vi "大富翁.vi"() -> ()   [LabVIEW 2014] (continued)
                      frame 4 {
                        n2785 = local read "玩家四財產"() -> (w2209:dbl)
                      }
                    }
                    n2786 = call "各種價格.vi"("Numeric"=w2178) -> ("買空地"=w2176:dbl)  [unwired: 4 in, 5 out]
                    n2787 = Greater Or Equal?(x=w2177, y=w2176) -> (x >= y?=w2175:bool)
                    n2788 = case shown="True" w2175 {
                      tunnel: w2178 -> [_ w2180]
                      frame False {
                        # "錢不夠"
                        n2789 = call "錢不夠.vi"() -> ()  [unwired: 4 in]
                      }
                      frame True {
                        # "錢夠"
                        n2790 = local read "換誰?"() -> (w2181:dbl)
                        n2791 = case shown="3" w2181 {
                          selector: w2181 -> [w2185 w2191 w2197 w2203]
                          tunnel: w2180 -> [w2184 w2190 w2196 w2202]
                          frame 1, Default {
                            # "誰買了地"
                            n2792 = call "各種價格.vi"("Numeric"=w2184) -> ("買空地"=w2183:dbl)  [unwired: 4 in, 5 out]
                            n2793 = local read "玩家一財產"() -> (w2187:dbl)
                            n2794 = Subtract(x=w2187, y=w2183) -> (x-y=w2186:dbl)
                            n2795 = local write "玩家一財產"(w2186) -> ()
                            n2796 = call "數字轉顏色.vi"("數字"=w2185) -> ("顏色數字"=w2182:dbl)  [unwired: 2 in]
                            n2797 = local write "17¾Á¤B"(w2182) -> ()
                            n2798 = local write "墾丁所有"(w2182) -> ()
                          }
                          frame 2 {
                            # "誰買了地"
                            n2799 = call "各種價格.vi"("Numeric"=w2190) -> ("買空地"=w2189:dbl)  [unwired: 4 in, 5 out]
                            n2800 = local read "玩家二財產"() -> (w2193:dbl)
                            n2801 = Subtract(x=w2193, y=w2189) -> (x-y=w2192:dbl)
                            n2802 = local write "玩家二財產"(w2192) -> ()
                            n2803 = call "數字轉顏色.vi"("數字"=w2191) -> ("顏色數字"=w2188:dbl)  [unwired: 2 in]
                            n2804 = local write "17¾Á¤B"(w2188) -> ()
                            n2805 = local write "墾丁所有"(w2188) -> ()
                          }
                          frame 3 {
                            # "誰買了地"
                            n2806 = local read "玩家三財產"() -> (w2198:dbl)
                            n2807 = call "各種價格.vi"("Numeric"=w2196) -> ("買空地"=w2195:dbl)  [unwired: 4 in, 5 out]
                            n2808 = Subtract(x=w2198, y=w2195) -> (x-y=w2199:dbl)
                            n2809 = call "數字轉顏色.vi"("數字"=w2197) -> ("顏色數字"=w2194:dbl)  [unwired: 2 in]
                            n2810 = local write "玩家三財產"(w2199) -> ()
                            n2811 = local write "17¾Á¤B"(w2194) -> ()
                            n2812 = local write "墾丁所有"(w2194) -> ()
                          }
                          frame 4 {
                            # "誰買了地"
                            n2813 = call "各種價格.vi"("Numeric"=w2202) -> ("買空地"=w2201:dbl)  [unwired: 4 in, 5 out]
                            n2814 = local read "玩家四財產"() -> (w2205:dbl)
                            n2815 = Subtract(x=w2205, y=w2201) -> (x-y=w2204:dbl)
                            n2816 = local write "玩家四財產"(w2204) -> ()
                            n2817 = call "數字轉顏色.vi"("數字"=w2203) -> ("顏色數字"=w2200:dbl)  [unwired: 2 in]
                            n2818 = local write "17¾Á¤B"(w2200) -> ()
                            n2819 = local write "墾丁所有"(w2200) -> ()
                          }
                        }
                      }
                    }
                  }
                }
              }
            }
          }
          frame 18 {
            n2820 = local read "屏東縣所有"() -> (w2210:u32)
            n2821 = Equal?(x=w2210, y=u32 16777215) -> (x = y?=w2213:bool)
            n2822 = case shown="True" w2213 {
              tunnel: w2212 -> [w2236 w2274]
              tunnel: [w2226 FALSE] -> w2211
              frame False {
                # "有主地"
                n2823 = local read "換誰?"() -> (w2229:dbl)
                n2824 = local read "屏東縣所有"() -> (w2217:u32)
                n2825 = call "數字轉顏色.vi"("數字"=w2229) -> ("顏色數字"=w2240:dbl)  [unwired: 2 in]
                n2826 = case shown="4" w2229 {
                  tunnel: [w2269 w2270 w2271 w2272] -> w2235
                  frame 1, Default {
                    n2827 = local read "玩家一財產"() -> (w2269:dbl)
                  }
                  frame 2 {
                    n2828 = local read "玩家二財產"() -> (w2270:dbl)
                  }
                  frame 3 {
                    n2829 = local read "玩家三財產"() -> (w2271:dbl)
                  }
                  frame 4 {
                    n2830 = local read "玩家四財產"() -> (w2272:dbl)
                  }
                }
                n2831 = Equal?(x=w2217, y=w2240) -> (x = y?=w2239:bool)
                n2832 = local read "18旅4"() -> (w2218:bool)
                n2833 = local read "18旅3"() -> (w2219:bool)
                n2834 = local read "18旅2"() -> (w2220:bool)
                n2835 = local read "18旅1"() -> (w2221:bool)
                n2836 = local read "18房4"() -> (w2222:bool)
                n2837 = local read "18房3"() -> (w2223:bool)
                n2838 = local read "18房2"() -> (w2224:bool)
                n2839 = local read "18房1"() -> (w2225:bool)
                n2840 = local read "屏東縣所有"() -> (w2216:u32)
                n2841 = call "房子數量.vi"("房子 1"=w2225, "房子 2"=w2224, "房子 3"=w2223, "房子 4"=w2222, "旅館 1"=w2221, "旅館 2"=w2220, "旅館 3"=w2219, "旅館 4"=w2218) -> ("房子數"=w2238:dbl, "旅館數"=w2237:dbl)  [unwired: 18 in]
                n2842 = call "顏色轉數字.vi"("顏色數字"=w2216) -> ("數字"=w2227:dbl)  [unwired: 2 in]
                n2843 = case shown="1, Default" w2227 {
                  tunnel: [w2245 w2246 w2247 w2248] -> w2231
                  frame 1, Default {
                    n2844 = local read "玩家一財產"() -> (w2245:dbl)
                  }
                  frame 2 {
                    n2845 = local read "玩家二財產"() -> (w2246:dbl)
                  }
                  frame 3 {
                    n2846 = local read "玩家三財產"() -> (w2247:dbl)
                  }
                  frame 4 {
                    n2847 = local read "玩家四財產"() -> (w2248:dbl)
                  }
                }
                n2848 = call "走到地.vi"("房子數量"=w2238, "自己的地?"=w2239, "旅館數量"=w2237, "編號"=w2236, "走到人財產"=w2235) -> ("走到人-?"=w2234:dbl, "蓋第幾棟"=w2232:dbl, "地主+?"=w2230:dbl, "破產?"=w2226:bool)
                n2849 = Subtract(x=w2235, y=w2234) -> (x-y=w2233:dbl)
                n2850 = Add(x=w2230, y=w2231) -> (x+y=w2228:dbl)
                n2851 = case shown="1, Default" w2227 {
                  tunnel: w2228 -> [w2241 w2242 w2243 w2244]
                  frame 1, Default {
                    n2852 = local write "玩家一財產"(w2241) -> ()
                  }
                  frame 2 {
                    n2853 = local write "玩家二財產"(w2242) -> ()
                  }
                  frame 3 {
                    n2854 = local write "玩家三財產"(w2243) -> ()
                  }
                  frame 4 {
                    n2855 = local write "玩家四財產"(w2244) -> ()
                  }
                }
                n2856 = case shown="6" w2232 {
                  frame 0, Default {
                  }
                  frame 1 {
                    n2857 = flat-sequence {
                      frame #0 {
                        n2858 = local write "18房1"(TRUE ("1房1")) -> ()
                      }
                      frame #1 {
                        n2859 = property on="18房1" class="Bool (strict)"("Visible"=TRUE) -> ()  [unwired: 2 in, 2 out]
                      }
                    }
                  }
                  frame 2 {
                    n2860 = flat-sequence {
                      frame #0 {
                        n2861 = local write "18房2"(TRUE ("1房2")) -> ()
                      }
                      frame #1 {
                        n2862 = property on="18房2" class="Bool (strict)"("Visible"=TRUE ("1房2")) -> ()  [unwired: 2 in, 2 out]
                      }
                    }
                  }
                  frame 3 {
                    n2863 = flat-sequence {
                      frame #0 {
                        n2864 = local write "18房3"(TRUE) -> ()
                      }
                      frame #1 {
                        n2865 = property on="18房3" class="Bool (strict)"("Visible"=TRUE) -> ()  [unwired: 2 in, 2 out]
                      }
                    }
                  }
                  frame 4 {
                    n2866 = flat-sequence {
                      frame #0 {
                        n2867 = local write "18房4"(TRUE) -> ()
                      }
                      frame #1 {
                        n2868 = property on="18房4" class="Bool (strict)"("Visible"=TRUE) -> ()  [unwired: 2 in, 2 out]
                      }
                    }
                  }
                  frame 5 {
                    n2869 = flat-sequence {
                      frame #0 {
                        n2870 = local write "18旅1"(TRUE) -> ()
                      }
                      frame #1 {
                        n2871 = property on="18旅1" class="Bool (strict)"("Visible"=TRUE) -> ()  [unwired: 2 in, 2 out]
                      }
                    }
                  }
                  frame 6 {
                    n2872 = flat-sequence {
                      frame #0 {
                        n2873 = local write "18旅2"(TRUE) -> ()
                      }
                      frame #1 {
                        n2874 = property on="18旅2" class="Bool (strict)"("Visible"=TRUE) -> ()  [unwired: 2 in, 2 out]
                      }
                    }
                  }
                  frame 7 {
                    n2875 = flat-sequence {
                      frame #0 {
                        n2876 = local write "18旅3"(TRUE) -> ()
                      }
                      frame #1 {
                        n2877 = property on="18旅3" class="Bool (strict)"("Visible"=TRUE) -> ()  [unwired: 2 in, 2 out]
                      }
                    }
                  }
                  frame 8 {
                    n2878 = flat-sequence {
                      frame #0 {
                        n2879 = local write "18旅4"(TRUE) -> ()
                      }
                      frame #1 {
                        n2880 = property on="18旅4" class="Bool (strict)"("Visible"=TRUE) -> ()  [unwired: 2 in, 2 out]
                      }
                    }
                  }
                }
                n2881 = case shown="1, Default" w2229 {
                  tunnel: w2233 -> [w2265 w2266 w2267 w2268]
                  frame 1, Default {
                    n2882 = local write "玩家一財產"(w2265) -> ()
                  }
                  frame 2 {
                    n2883 = local write "玩家二財產"(w2266) -> ()
                  }
                  frame 3 {
                    n2884 = local write "玩家三財產"(w2267) -> ()
                  }
                  frame 4 {
                    n2885 = local write "玩家四財產"(w2268) -> ()
                  }
                }
              }
              frame True {
                # "無主地"
                n2886 = call "購買土地.vi"() -> ("確定 2"=w2275:bool)  [unwired: 3 in]
                n2887 = case shown="True" w2275 {
                  tunnel: w2274 -> [_ w2279]
                  frame False {
                    # "不買"
                  }
                  frame True {
                    # "要買"
                    n2888 = local read "換誰?"() -> (w2280:dbl)
                    n2889 = case shown="4" w2280 {
                      tunnel: [w2307 w2308 w2309 w2310] -> w2278
                      frame 1, Default {
                        n2890 = local read "玩家一財產"() -> (w2307:dbl)
                      }
                      frame 2 {
                        n2891 = local read "玩家二財產"() -> (w2308:dbl)
                      }
                      frame 3 {
                        n2892 = local read "玩家三財產"() -> (w2309:dbl)
                      }
                      frame 4 {
                        n2893 = local read "玩家四財產"() -> (w2310:dbl)
                      }
                    }
                    n2894 = call "各種價格.vi"("Numeric"=w2279) -> ("買空地"=w2277:dbl)  [unwired: 4 in, 5 out]
                    n2895 = Greater Or Equal?(x=w2278, y=w2277) -> (x >= y?=w2276:bool)
                    n2896 = case shown="True" w2276 {
                      tunnel: w2279 -> [_ w2281]
                      frame False {
                        # "錢不夠"
                        n2897 = call "錢不夠.vi"() -> ()  [unwired: 4 in]
                      }
                      frame True {
                        # "錢夠"
                        n2898 = local read "換誰?"() -> (w2282:dbl)
                        n2899 = case shown="1, Default" w2282 {
                          selector: w2282 -> [w2286 w2292 w2298 w2304]
                          tunnel: w2281 -> [w2285 w2291 w2297 w2303]
                          frame 1, Default {
                            # "誰買了地"
                            n2900 = call "各種價格.vi"("Numeric"=w2285) -> ("買空地"=w2284:dbl)  [unwired: 4 in, 5 out]
                            n2901 = local read "玩家一財產"() -> (w2288:dbl)
                            n2902 = Subtract(x=w2288, y=w2284) -> (x-y=w2287:dbl)
                            n2903 = local write "玩家一財產"(w2287) -> ()
                            n2904 = call "數字轉顏色.vi"("數字"=w2286) -> ("顏色數字"=w2283:dbl)  [unwired: 2 in]
                            n2905 = local write "18屏東縣"(w2283) -> ()
                            n2906 = local write "屏東縣所有"(w2283) -> ()
                          }
                          frame 2 {
                            # "誰買了地"
                            n2907 = call "各種價格.vi"("Numeric"=w2291) -> ("買空地"=w2290:dbl)  [unwired: 4 in, 5 out]
                            n2908 = local read "玩家二財產"() -> (w2294:dbl)
                            n2909 = Subtract(x=w2294, y=w2290) -> (x-y=w2293:dbl)
                            n2910 = local write "玩家二財產"(w2293) -> ()
                            n2911 = call "數字轉顏色.vi"("數字"=w2292) -> ("顏色數字"=w2289:dbl)  [unwired: 2 in]
                            n2912 = local write "18屏東縣"(w2289) -> ()
                            n2913 = local write "屏東縣所有"(w2289) -> ()
                          }
                          frame 3 {
                            # "誰買了地"
                            n2914 = local read "玩家三財產"() -> (w2299:dbl)
                            n2915 = call "各種價格.vi"("Numeric"=w2297) -> ("買空地"=w2296:dbl)  [unwired: 4 in, 5 out]
                            n2916 = Subtract(x=w2299, y=w2296) -> (x-y=w2300:dbl)
                            n2917 = call "數字轉顏色.vi"("數字"=w2298) -> ("顏色數字"=w2295:dbl)  [unwired: 2 in]
                            n2918 = local write "玩家三財產"(w2300) -> ()
                            n2919 = local write "18屏東縣"(w2295) -> ()
                            n2920 = local write "屏東縣所有"(w2295) -> ()
                          }
                          frame 4 {
                            # "誰買了地"
                            n2921 = call "各種價格.vi"("Numeric"=w2303) -> ("買空地"=w2302:dbl)  [unwired: 4 in, 5 out]
                            n2922 = local read "玩家四財產"() -> (w2306:dbl)
                            n2923 = Subtract(x=w2306, y=w2302) -> (x-y=w2305:dbl)
                            n2924 = local write "玩家四財產"(w2305) -> ()
                            n2925 = call "數字轉顏色.vi"("數字"=w2304) -> ("顏色數字"=w2301:dbl)  [unwired: 2 in]
                            n2926 = local write "18屏東縣"(w2301) -> ()
                            n2927 = local write "屏東縣所有"(w2301) -> ()
                          }
                        }
                      }
                    }
                  }
                }
              }
            }
          }
          frame 19 {
            # "公園"
            n2928 = call "19公園.vi"() -> ()  [unwired: 4 in]
          }
          frame 20 {
            n2929 = local read "高雄市所有"() -> (w2313:u32)
            n2930 = Equal?(x=w2313, y=u32 16777215) -> (x = y?=w2316:bool)
            n2931 = case shown="False" w2316 {
              tunnel: w2315 -> [w2339 w2377]
              tunnel: [w2329 FALSE] -> w2314
              frame False {
                # "有主地"
                n2932 = local read "換誰?"() -> (w2332:dbl)
                n2933 = local read "高雄市所有"() -> (w2320:u32)
                n2934 = call "數字轉顏色.vi"("數字"=w2332) -> ("顏色數字"=w2343:dbl)  [unwired: 2 in]
                n2935 = case shown="4" w2332 {
                  tunnel: [w2372 w2373 w2374 w2375] -> w2338
                  frame 1, Default {
                    n2936 = local read "玩家一財產"() -> (w2372:dbl)
                  }
                  frame 2 {
                    n2937 = local read "玩家二財產"() -> (w2373:dbl)
                  }
                  frame 3 {
                    n2938 = local read "玩家三財產"() -> (w2374:dbl)
                  }
                  frame 4 {
                    n2939 = local read "玩家四財產"() -> (w2375:dbl)
                  }
                }
                n2940 = Equal?(x=w2320, y=w2343) -> (x = y?=w2342:bool)
                n2941 = local read "20旅4"() -> (w2321:bool)
                n2942 = local read "20旅3"() -> (w2322:bool)
                n2943 = local read "20旅2"() -> (w2323:bool)
                n2944 = local read "20旅1"() -> (w2324:bool)
                n2945 = local read "20房4"() -> (w2325:bool)
                n2946 = local read "20房3"() -> (w2326:bool)
                n2947 = local read "20房2"() -> (w2327:bool)
                n2948 = local read "20房1"() -> (w2328:bool)
                n2949 = local read "高雄市所有"() -> (w2319:u32)
                n2950 = call "房子數量.vi"("房子 1"=w2328, "房子 2"=w2327, "房子 3"=w2326, "房子 4"=w2325, "旅館 1"=w2324, "旅館 2"=w2323, "旅館 3"=w2322, "旅館 4"=w2321) -> ("房子數"=w2341:dbl, "旅館數"=w2340:dbl)  [unwired: 18 in]
                n2951 = call "顏色轉數字.vi"("顏色數字"=w2319) -> ("數字"=w2330:dbl)  [unwired: 2 in]
                n2952 = case shown="1, Default" w2330 {
                  tunnel: [w2348 w2349 w2350 w2351] -> w2334
                  frame 1, Default {
                    n2953 = local read "玩家一財產"() -> (w2348:dbl)
                  }
                  frame 2 {
                    n2954 = local read "玩家二財產"() -> (w2349:dbl)
                  }
                  frame 3 {
                    n2955 = local read "玩家三財產"() -> (w2350:dbl)
                  }
                  frame 4 {
                    n2956 = local read "玩家四財產"() -> (w2351:dbl)
                  }
                }
                n2957 = call "走到地.vi"("房子數量"=w2341, "自己的地?"=w2342, "旅館數量"=w2340, "編號"=w2339, "走到人財產"=w2338) -> ("走到人-?"=w2337:dbl, "蓋第幾棟"=w2335:dbl, "地主+?"=w2333:dbl, "破產?"=w2329:bool)
                n2958 = Subtract(x=w2338, y=w2337) -> (x-y=w2336:dbl)
                n2959 = Add(x=w2333, y=w2334) -> (x+y=w2331:dbl)
                n2960 = case shown="1, Default" w2330 {
                  tunnel: w2331 -> [w2344 w2345 w2346 w2347]
                  frame 1, Default {
                    n2961 = local write "玩家一財產"(w2344) -> ()
                  }
                  frame 2 {
                    n2962 = local write "玩家二財產"(w2345) -> ()
                  }
                  frame 3 {
                    n2963 = local write "玩家三財產"(w2346) -> ()
                  }
                  frame 4 {
                    n2964 = local write "玩家四財產"(w2347) -> ()
                  }
                }
                n2965 = case shown="7" w2335 {
                  frame 0, Default {
                  }
                  frame 1 {
                    n2966 = flat-sequence {
                      frame #0 {
                        n2967 = local write "20房1"(TRUE ("1房1")) -> ()
                      }
                      frame #1 {
                        n2968 = property on="20房1" class="Bool (strict)"("Visible"=TRUE) -> ()  [unwired: 2 in, 2 out]
                      }
                    }
                  }
                  frame 2 {
                    n2969 = flat-sequence {
                      frame #0 {
                        n2970 = local write "20房2"(TRUE ("1房2")) -> ()
                      }
                      frame #1 {
                        n2971 = property on="20房2" class="Bool (strict)"("Visible"=TRUE ("1房2")) -> ()  [unwired: 2 in, 2 out]
                      }
                    }
                  }
                  frame 3 {
                    n2972 = flat-sequence {
                      frame #0 {
                        n2973 = local write "20房3"(TRUE) -> ()
                      }
                      frame #1 {
                        n2974 = property on="20房3" class="Bool (strict)"("Visible"=TRUE) -> ()  [unwired: 2 in, 2 out]
                      }
                    }
                  }
                  frame 4 {
                    n2975 = flat-sequence {
                      frame #0 {
                        n2976 = local write "20房4"(TRUE) -> ()
                      }
                      frame #1 {
                        n2977 = property on="20房4" class="Bool (strict)"("Visible"=TRUE) -> ()  [unwired: 2 in, 2 out]
                      }
                    }
                  }
                  frame 5 {
                    n2978 = flat-sequence {
                      frame #0 {
                        n2979 = local write "20旅1"(TRUE) -> ()
                      }
                      frame #1 {
                        n2980 = property on="20旅1" class="Bool (strict)"("Visible"=TRUE) -> ()  [unwired: 2 in, 2 out]
                      }
                    }
                  }
                  frame 6 {
                    n2981 = flat-sequence {
                      frame #0 {
                        n2982 = local write "20旅2"(TRUE) -> ()
                      }
                      frame #1 {
                        n2983 = property on="20旅2" class="Bool (strict)"("Visible"=TRUE) -> ()  [unwired: 2 in, 2 out]
                      }
                    }
                  }
                  frame 7 {
                    n2984 = flat-sequence {
                      frame #0 {
                        n2985 = local write "20旅3"(TRUE) -> ()
                      }
                      frame #1 {
                        n2986 = property on="20旅3" class="Bool (strict)"("Visible"=TRUE) -> ()  [unwired: 2 in, 2 out]
                      }
                    }
                  }
                  frame 8 {
                    n2987 = flat-sequence {
                      frame #0 {
                        n2988 = local write "20旅4"(TRUE) -> ()
                      }
                      frame #1 {
                        n2989 = property on="20旅4" class="Bool (strict)"("Visible"=TRUE) -> ()  [unwired: 2 in, 2 out]
                      }
                    }
                  }
                }
                n2990 = case shown="1, Default" w2332 {
                  tunnel: w2336 -> [w2368 w2369 w2370 w2371]
                  frame 1, Default {
                    n2991 = local write "玩家一財產"(w2368) -> ()
                  }
                  frame 2 {
                    n2992 = local write "玩家二財產"(w2369) -> ()
                  }
                  frame 3 {
                    n2993 = local write "玩家三財產"(w2370) -> ()
                  }
                  frame 4 {
                    n2994 = local write "玩家四財產"(w2371) -> ()
                  }
                }
              }
              frame True {
                # "無主地"
                n2995 = call "購買土地.vi"() -> ("確定 2"=w2378:bool)  [unwired: 3 in]
                n2996 = case shown="True" w2378 {
                  tunnel: w2377 -> [_ w2382]
                  frame False {
                    # "不買"
                  }
                  frame True {
                    # "要買"
                    n2997 = local read "換誰?"() -> (w2383:dbl)
                    n2998 = case shown="4" w2383 {
                      tunnel: [w2410 w2411 w2412 w2413] -> w2381
                      frame 1, Default {
                        n2999 = local read "玩家一財產"() -> (w2410:dbl)
                      }
                      frame 2 {
                        n3000 = local read "玩家二財產"() -> (w2411:dbl)
                      }
                      frame 3 {
                        n3001 = local read "玩家三財產"() -> (w2412:dbl)
                      }
                      frame 4 {
                        n3002 = local read "玩家四財產"() -> (w2413:dbl)
                      }
                    }
                    n3003 = call "各種價格.vi"("Numeric"=w2382) -> ("買空地"=w2380:dbl)  [unwired: 4 in, 5 out]
                    n3004 = Greater Or Equal?(x=w2381, y=w2380) -> (x >= y?=w2379:bool)
                    n3005 = case shown="True" w2379 {
                      tunnel: w2382 -> [_ w2384]
                      frame False {
                        # "錢不夠"
                        n3006 = call "錢不夠.vi"() -> ()  [unwired: 4 in]
                      }
                      frame True {
                        # "錢夠"
                        n3007 = local read "換誰?"() -> (w2385:dbl)
                        n3008 = case shown="3" w2385 {
                          selector: w2385 -> [w2389 w2395 w2401 w2407]
                          tunnel: w2384 -> [w2388 w2394 w2400 w2406]
                          frame 1, Default {
                            # "誰買了地"
                            n3009 = call "各種價格.vi"("Numeric"=w2388) -> ("買空地"=w2387:dbl)  [unwired: 4 in, 5 out]
                            n3010 = local read "玩家一財產"() -> (w2391:dbl)
                            n3011 = Subtract(x=w2391, y=w2387) -> (x-y=w2390:dbl)
                            n3012 = local write "玩家一財產"(w2390) -> ()
                            n3013 = call "數字轉顏色.vi"("數字"=w2389) -> ("顏色數字"=w2386:dbl)  [unwired: 2 in]
                            n3014 = local write "20高雄市"(w2386) -> ()
                            n3015 = local write "高雄市所有"(w2386) -> ()
                          }
                          frame 2 {
                            # "誰買了地"
                            n3016 = call "各種價格.vi"("Numeric"=w2394) -> ("買空地"=w2393:dbl)  [unwired: 4 in, 5 out]
                            n3017 = local read "玩家二財產"() -> (w2397:dbl)
                            n3018 = Subtract(x=w2397, y=w2393) -> (x-y=w2396:dbl)
                            n3019 = local write "玩家二財產"(w2396) -> ()
                            n3020 = call "數字轉顏色.vi"("數字"=w2395) -> ("顏色數字"=w2392:dbl)  [unwired: 2 in]
                            n3021 = local write "20高雄市"(w2392) -> ()
                            n3022 = local write "高雄市所有"(w2392) -> ()
                          }
                          frame 3 {
                            # "誰買了地"
                            n3023 = local read "玩家三財產"() -> (w2402:dbl)
                            n3024 = call "各種價格.vi"("Numeric"=w2400) -> ("買空地"=w2399:dbl)  [unwired: 4 in, 5 out]
                            n3025 = Subtract(x=w2402, y=w2399) -> (x-y=w2403:dbl)
                            n3026 = call "數字轉顏色.vi"("數字"=w2401) -> ("顏色數字"=w2398:dbl)  [unwired: 2 in]
                            n3027 = local write "玩家三財產"(w2403) -> ()
                            n3028 = local write "20高雄市"(w2398) -> ()
                            n3029 = local write "高雄市所有"(w2398) -> ()
                          }
                          frame 4 {
                            # "誰買了地"
                            n3030 = call "各種價格.vi"("Numeric"=w2406) -> ("買空地"=w2405:dbl)  [unwired: 4 in, 5 out]
                            n3031 = local read "玩家四財產"() -> (w2409:dbl)
                            n3032 = Subtract(x=w2409, y=w2405) -> (x-y=w2408:dbl)
                            n3033 = local write "玩家四財產"(w2408) -> ()
                            n3034 = call "數字轉顏色.vi"("數字"=w2407) -> ("顏色數字"=w2404:dbl)  [unwired: 2 in]
                            n3035 = local write "20高雄市"(w2404) -> ()
                            n3036 = local write "高雄市所有"(w2404) -> ()
                          }
                        }
                      }
                    }
                  }
                }
              }
            }
          }
          frame 21 {
            n3037 = local read "台南市所有"() -> (w2414:u32)
            n3038 = Equal?(x=w2414, y=u32 16777215) -> (x = y?=w2417:bool)
            n3039 = case shown="True" w2417 {
              tunnel: w2416 -> [w2440 w2478]
              tunnel: [w2430 FALSE] -> w2415
              frame False {
                # "有主地"
                n3040 = local read "換誰?"() -> (w2433:dbl)
                n3041 = local read "台南市所有"() -> (w2421:u32)
                n3042 = call "數字轉顏色.vi"("數字"=w2433) -> ("顏色數字"=w2444:dbl)  [unwired: 2 in]
                n3043 = case shown="4" w2433 {
                  tunnel: [w2473 w2474 w2475 w2476] -> w2439
                  frame 1, Default {
                    n3044 = local read "玩家一財產"() -> (w2473:dbl)
                  }
                  frame 2 {
                    n3045 = local read "玩家二財產"() -> (w2474:dbl)
                  }
                  frame 3 {
                    n3046 = local read "玩家三財產"() -> (w2475:dbl)
                  }
                  frame 4 {
                    n3047 = local read "玩家四財產"() -> (w2476:dbl)
                  }
                }
                n3048 = Equal?(x=w2421, y=w2444) -> (x = y?=w2443:bool)
                n3049 = local read "21旅4"() -> (w2429:bool)
                n3050 = local read "21旅3"() -> (w2428:bool)
                n3051 = local read "21旅2"() -> (w2427:bool)
                n3052 = local read "21旅1"() -> (w2426:bool)
                n3053 = local read "21房4"() -> (w2425:bool)
                n3054 = local read "21房3"() -> (w2424:bool)
                n3055 = local read "21房2"() -> (w2423:bool)
                n3056 = local read "21房1"() -> (w2422:bool)
                n3057 = local read "台南市所有"() -> (w2420:u32)
                n3058 = call "房子數量.vi"("房子 1"=w2422, "房子 2"=w2423, "房子 3"=w2424, "房子 4"=w2425, "旅館 1"=w2426, "旅館 2"=w2427, "旅館 3"=w2428, "旅館 4"=w2429) -> ("房子數"=w2442:dbl, "旅館數"=w2441:dbl)  [unwired: 18 in]
                n3059 = call "顏色轉數字.vi"("顏色數字"=w2420) -> ("數字"=w2431:dbl)  [unwired: 2 in]
                n3060 = case shown="1, Default" w2431 {
                  tunnel: [w2449 w2450 w2451 w2452] -> w2435
                  frame 1, Default {
                    n3061 = local read "玩家一財產"() -> (w2449:dbl)
                  }
                  frame 2 {
                    n3062 = local read "玩家二財產"() -> (w2450:dbl)
                  }
                  frame 3 {
                    n3063 = local read "玩家三財產"() -> (w2451:dbl)
                  }
                  frame 4 {
                    n3064 = local read "玩家四財產"() -> (w2452:dbl)
                  }
                }
                n3065 = call "走到地.vi"("房子數量"=w2442, "自己的地?"=w2443, "旅館數量"=w2441, "編號"=w2440, "走到人財產"=w2439) -> ("走到人-?"=w2438:dbl, "蓋第幾棟"=w2436:dbl, "地主+?"=w2434:dbl, "破產?"=w2430:bool)
                n3066 = Subtract(x=w2439, y=w2438) -> (x-y=w2437:dbl)
                n3067 = Add(x=w2434, y=w2435) -> (x+y=w2432:dbl)
                n3068 = case shown="1, Default" w2431 {
                  tunnel: w2432 -> [w2445 w2446 w2447 w2448]
                  frame 1, Default {
                    n3069 = local write "玩家一財產"(w2445) -> ()
                  }
                  frame 2 {
                    n3070 = local write "玩家二財產"(w2446) -> ()
                  }
                  frame 3 {
                    n3071 = local write "玩家三財產"(w2447) -> ()
                  }
                  frame 4 {
                    n3072 = local write "玩家四財產"(w2448) -> ()
                  }
                }
                n3073 = case shown="3" w2436 {
                  frame 0, Default {
                  }
                  frame 1 {
                    n3074 = flat-sequence {
                      frame #0 {
                        n3075 = local write "21房1"(TRUE ("1房1")) -> ()
                      }
                      frame #1 {
                        n3076 = property on="21房1" class="Bool (strict)"("Visible"=TRUE) -> ()  [unwired: 2 in, 2 out]
                      }
                    }
                  }
                  frame 2 {
                    n3077 = flat-sequence {
                      frame #0 {
                        n3078 = local write "21房2"(TRUE ("1房2")) -> ()
                      }
                      frame #1 {
                        n3079 = property on="21房2" class="Bool (strict)"("Visible"=TRUE ("1房2")) -> ()  [unwired: 2 in, 2 out]
                      }
                    }
                  }
                  frame 3 {
                    n3080 = flat-sequence {
                      frame #0 {
                        n3081 = local write "21房3"(TRUE) -> ()
                      }
                      frame #1 {
                        n3082 = property on="21房3" class="Bool (strict)"("Visible"=TRUE) -> ()  [unwired: 2 in, 2 out]
                      }
                    }
                  }
                  frame 4 {
                    n3083 = flat-sequence {
                      frame #0 {
                        n3084 = local write "21房4"(TRUE) -> ()
                      }
                      frame #1 {
                        n3085 = property on="21房4" class="Bool (strict)"("Visible"=TRUE) -> ()  [unwired: 2 in, 2 out]
                      }
                    }
                  }
                  frame 5 {
                    n3086 = flat-sequence {
                      frame #0 {
                        n3087 = local write "21旅1"(TRUE) -> ()
                      }
                      frame #1 {
                        n3088 = property on="21旅1" class="Bool (strict)"("Visible"=TRUE) -> ()  [unwired: 2 in, 2 out]
                      }
                    }
                  }
                  frame 6 {
                    n3089 = flat-sequence {
                      frame #0 {
                        n3090 = local write "21旅2"(TRUE) -> ()
                      }
                      frame #1 {
                        n3091 = property on="21旅2" class="Bool (strict)"("Visible"=TRUE) -> ()  [unwired: 2 in, 2 out]
                      }
                    }
                  }
                  frame 7 {
                    n3092 = flat-sequence {
                      frame #0 {
                        n3093 = local write "21旅3"(TRUE) -> ()
                      }
                      frame #1 {
                        n3094 = property on="21旅3" class="Bool (strict)"("Visible"=TRUE) -> ()  [unwired: 2 in, 2 out]
                      }
                    }
                  }
                  frame 8 {
                    n3095 = flat-sequence {
                      frame #0 {
                        n3096 = local write "21旅4"(TRUE) -> ()
                      }
                      frame #1 {
                        n3097 = property on="21旅4" class="Bool (strict)"("Visible"=TRUE) -> ()  [unwired: 2 in, 2 out]
                      }
                    }
                  }
                }
                n3098 = case shown="1, Default" w2433 {
                  tunnel: w2437 -> [w2469 w2470 w2471 w2472]
                  frame 1, Default {
                    n3099 = local write "玩家一財產"(w2469) -> ()
                  }
                  frame 2 {
                    n3100 = local write "玩家二財產"(w2470) -> ()
                  }
                  frame 3 {
                    n3101 = local write "玩家三財產"(w2471) -> ()
                  }
                  frame 4 {
                    n3102 = local write "玩家四財產"(w2472) -> ()
                  }
                }
              }
              frame True {
                # "無主地"
                n3103 = call "購買土地.vi"() -> ("確定 2"=w2479:bool)  [unwired: 3 in]
                n3104 = case shown="True" w2479 {
                  tunnel: w2478 -> [_ w2483]
                  frame False {
                    # "不買"
                  }
                  frame True {
                    # "要買"
                    n3105 = local read "換誰?"() -> (w2484:dbl)
                    n3106 = case shown="4" w2484 {
                      tunnel: [w2511 w2512 w2513 w2514] -> w2482
                      frame 1, Default {
                        n3107 = local read "玩家一財產"() -> (w2511:dbl)
                      }
                      frame 2 {
                        n3108 = local read "玩家二財產"() -> (w2512:dbl)
                      }
                      frame 3 {
                        n3109 = local read "玩家三財產"() -> (w2513:dbl)
                      }
                      frame 4 {
                        n3110 = local read "玩家四財產"() -> (w2514:dbl)
                      }
                    }
                    n3111 = call "各種價格.vi"("Numeric"=w2483) -> ("買空地"=w2481:dbl)  [unwired: 4 in, 5 out]
                    n3112 = Greater Or Equal?(x=w2482, y=w2481) -> (x >= y?=w2480:bool)
                    n3113 = case shown="True" w2480 {
                      tunnel: w2483 -> [_ w2485]
                      frame False {
                        # "錢不夠"
                        n3114 = call "錢不夠.vi"() -> ()  [unwired: 4 in]
                      }
                      frame True {
                        # "錢夠"
                        n3115 = local read "換誰?"() -> (w2486:dbl)
                        n3116 = case shown="3" w2486 {
                          selector: w2486 -> [w2490 w2496 w2502 w2508]
                          tunnel: w2485 -> [w2489 w2495 w2501 w2507]
                          frame 1, Default {
                            # "誰買了地"
                            n3117 = call "各種價格.vi"("Numeric"=w2489) -> ("買空地"=w2488:dbl)  [unwired: 4 in, 5 out]
                            n3118 = local read "玩家一財產"() -> (w2492:dbl)
                            n3119 = Subtract(x=w2492, y=w2488) -> (x-y=w2491:dbl)
                            n3120 = local write "玩家一財產"(w2491) -> ()
                            n3121 = call "數字轉顏色.vi"("數字"=w2490) -> ("顏色數字"=w2487:dbl)  [unwired: 2 in]
                            n3122 = local write "21台南市"(w2487) -> ()
                            n3123 = local write "台南市所有"(w2487) -> ()
                          }
                          frame 2 {
                            # "誰買了地"
                            n3124 = call "各種價格.vi"("Numeric"=w2495) -> ("買空地"=w2494:dbl)  [unwired: 4 in, 5 out]
                            n3125 = local read "玩家二財產"() -> (w2498:dbl)
                            n3126 = Subtract(x=w2498, y=w2494) -> (x-y=w2497:dbl)
                            n3127 = local write "玩家二財產"(w2497) -> ()
                            n3128 = call "數字轉顏色.vi"("數字"=w2496) -> ("顏色數字"=w2493:dbl)  [unwired: 2 in]
                            n3129 = local write "21台南市"(w2493) -> ()
                            n3130 = local write "台南市所有"(w2493) -> ()
                          }
                          frame 3 {
                            # "誰買了地"
                            n3131 = local read "玩家三財產"() -> (w2503:dbl)
                            n3132 = call "各種價格.vi"("Numeric"=w2501) -> ("買空地"=w2500:dbl)  [unwired: 4 in, 5 out]
                            n3133 = Subtract(x=w2503, y=w2500) -> (x-y=w2504:dbl)
                            n3134 = call "數字轉顏色.vi"("數字"=w2502) -> ("顏色數字"=w2499:dbl)  [unwired: 2 in]
                            n3135 = local write "玩家三財產"(w2504) -> ()
                            n3136 = local write "21台南市"(w2499) -> ()
                            n3137 = local write "台南市所有"(w2499) -> ()
                          }
                          frame 4 {
                            # "誰買了地"
                            n3138 = call "各種價格.vi"("Numeric"=w2507) -> ("買空地"=w2506:dbl)  [unwired: 4 in, 5 out]
                            n3139 = local read "玩家四財產"() -> (w2510:dbl)
                            n3140 = Subtract(x=w2510, y=w2506) -> (x-y=w2509:dbl)
                            n3141 = local write "玩家四財產"(w2509) -> ()
                            n3142 = call "數字轉顏色.vi"("數字"=w2508) -> ("顏色數字"=w2505:dbl)  [unwired: 2 in]
                            n3143 = local write "21台南市"(w2505) -> ()
                            n3144 = local write "台南市所有"(w2505) -> ()
                          }
                        }
                      }
                    }
                  }
                }
              }
            }
          }
          frame 22 {
            n3145 = local read "阿里山所有"() -> (w2515:u32)
            n3146 = Equal?(x=w2515, y=u32 16777215) -> (x = y?=w2518:bool)
            n3147 = case shown="True" w2518 {
              tunnel: w2517 -> [w2541 w2579]
              tunnel: [w2531 FALSE] -> w2516
              frame False {
                # "有主地"
                n3148 = local read "換誰?"() -> (w2534:dbl)
                n3149 = local read "阿里山所有"() -> (w2521:u32)
                n3150 = call "數字轉顏色.vi"("數字"=w2534) -> ("顏色數字"=w2545:dbl)  [unwired: 2 in]
                n3151 = local read "阿里山所有"() -> (w2522:u32)
                n3152 = case shown="4" w2534 {
                  tunnel: [w2574 w2575 w2576 w2577] -> w2540
                  frame 1, Default {
                    n3153 = local read "玩家一財產"() -> (w2574:dbl)
                  }
                  frame 2 {
                    n3154 = local read "玩家二財產"() -> (w2575:dbl)
                  }
                  frame 3 {
                    n3155 = local read "玩家三財產"() -> (w2576:dbl)
                  }
                  frame 4 {
                    n3156 = local read "玩家四財產"() -> (w2577:dbl)
                  }
                }
                n3157 = Equal?(x=w2521, y=w2545) -> (x = y?=w2544:bool)
                n3158 = local read "22旅4"() -> (w2523:bool)
                n3159 = local read "22旅3"() -> (w2524:bool)
                n3160 = local read "22旅2"() -> (w2525:bool)
                n3161 = local read "22旅1"() -> (w2526:bool)
                n3162 = local read "22房4"() -> (w2527:bool)
                n3163 = local read "22房3"() -> (w2528:bool)
                n3164 = local read "22房2"() -> (w2529:bool)
                n3165 = local read "22房1"() -> (w2530:bool)
                n3166 = call "房子數量.vi"("房子 1"=w2530, "房子 2"=w2529, "房子 3"=w2528, "房子 4"=w2527, "旅館 1"=w2526, "旅館 2"=w2525, "旅館 3"=w2524, "旅館 4"=w2523) -> ("房子數"=w2543:dbl, "旅館數"=w2542:dbl)  [unwired: 18 in]
                n3167 = call "顏色轉數字.vi"("顏色數字"=w2522) -> ("數字"=w2532:dbl)  [unwired: 2 in]
                n3168 = case shown="1, Default" w2532 {
                  tunnel: [w2550 w2551 w2552 w2553] -> w2536
                  frame 1, Default {
                    n3169 = local read "玩家一財產"() -> (w2550:dbl)
                  }
                  frame 2 {
                    n3170 = local read "玩家二財產"() -> (w2551:dbl)
                  }
                  frame 3 {
                    n3171 = local read "玩家三財產"() -> (w2552:dbl)
                  }
                  frame 4 {
                    n3172 = local read "玩家四財產"() -> (w2553:dbl)
                  }
                }
                n3173 = call "走到地.vi"("房子數量"=w2543, "自己的地?"=w2544, "旅館數量"=w2542, "編號"=w2541, "走到人財產"=w2540) -> ("走到人-?"=w2539:dbl, "蓋第幾棟"=w2537:dbl, "地主+?"=w2535:dbl, "破產?"=w2531:bool)
                n3174 = Subtract(x=w2540, y=w2539) -> (x-y=w2538:dbl)
                n3175 = Add(x=w2535, y=w2536) -> (x+y=w2533:dbl)
                n3176 = case shown="1, Default" w2532 {
                  tunnel: w2533 -> [w2546 w2547 w2548 w2549]
                  frame 1, Default {
                    n3177 = local write "玩家一財產"(w2546) -> ()
                  }
                  frame 2 {
                    n3178 = local write "玩家二財產"(w2547) -> ()
                  }
                  frame 3 {
                    n3179 = local write "玩家三財產"(w2548) -> ()
                  }
                  frame 4 {
                    n3180 = local write "玩家四財產"(w2549) -> ()
                  }
                }
                n3181 = case shown="8" w2537 {
                  frame 0, Default {
                  }
                  frame 1 {
                    n3182 = flat-sequence {
                      frame #0 {
                        n3183 = local write "22房1"(TRUE ("1房1")) -> ()
                      }
                      frame #1 {
                        n3184 = property on="22房1" class="Bool (strict)"("Visible"=TRUE) -> ()  [unwired: 2 in, 2 out]
                      }
                    }
                  }
                  frame 2 {
                    n3185 = flat-sequence {
                      frame #0 {
                        n3186 = local write "22房2"(TRUE ("1房2")) -> ()
                      }
                      frame #1 {
                        n3187 = property on="22房2" class="Bool (strict)"("Visible"=TRUE ("1房2")) -> ()  [unwired: 2 in, 2 out]
                      }
                    }
                  }
                  frame 3 {
                    n3188 = flat-sequence {
                      frame #0 {
                        n3189 = local write "22房3"(TRUE) -> ()
                      }
                      frame #1 {
                        n3190 = property on="22房3" class="Bool (strict)"("Visible"=TRUE) -> ()  [unwired: 2 in, 2 out]
                      }
                    }
                  }
                  frame 4 {
                    n3191 = flat-sequence {
                      frame #0 {
                        n3192 = local write "22房4"(TRUE) -> ()
                      }
                      frame #1 {
                        n3193 = property on="22房4" class="Bool (strict)"("Visible"=TRUE) -> ()  [unwired: 2 in, 2 out]
                      }
                    }
                  }
                  frame 5 {
                    n3194 = flat-sequence {
                      frame #0 {
                        n3195 = local write "22旅1"(TRUE) -> ()
                      }
                      frame #1 {
                        n3196 = property on="22旅1" class="Bool (strict)"("Visible"=TRUE) -> ()  [unwired: 2 in, 2 out]
                      }
                    }
                  }
                  frame 6 {
                    n3197 = flat-sequence {
                      frame #0 {
                        n3198 = local write "22旅2"(TRUE) -> ()
                      }
                      frame #1 {
                        n3199 = property on="22旅2" class="Bool (strict)"("Visible"=TRUE) -> ()  [unwired: 2 in, 2 out]
                      }
                    }
                  }
                  frame 7 {
                    n3200 = flat-sequence {
                      frame #0 {
                        n3201 = local write "22旅3"(TRUE) -> ()
                      }
                      frame #1 {
                        n3202 = property on="22旅3" class="Bool (strict)"("Visible"=TRUE) -> ()  [unwired: 2 in, 2 out]
                      }
                    }
                  }
                  frame 8 {
                    n3203 = flat-sequence {
                      frame #0 {
                        n3204 = local write "22旅4"(TRUE) -> ()
                      }
                      frame #1 {
                        n3205 = property on="22旅4" class="Bool (strict)"("Visible"=TRUE) -> ()  [unwired: 2 in, 2 out]
                      }
                    }
                  }
                }
                n3206 = case shown="1, Default" w2534 {
                  tunnel: w2538 -> [w2570 w2571 w2572 w2573]
                  frame 1, Default {
                    n3207 = local write "玩家一財產"(w2570) -> ()
                  }
                  frame 2 {
                    n3208 = local write "玩家二財產"(w2571) -> ()
                  }
                  frame 3 {
                    n3209 = local write "玩家三財產"(w2572) -> ()
                  }
                  frame 4 {
                    n3210 = local write "玩家四財產"(w2573) -> ()
                  }
                }
              }
              frame True {
                # "無主地"
                n3211 = call "購買土地.vi"() -> ("確定 2"=w2580:bool)  [unwired: 3 in]
                n3212 = case shown="True" w2580 {
                  tunnel: w2579 -> [_ w2584]
                  frame False {
                    # "不買"
                  }
                  frame True {
                    # "要買"
                    n3213 = local read "換誰?"() -> (w2585:dbl)
                    n3214 = case shown="4" w2585 {
                      tunnel: [w2612 w2613 w2614 w2615] -> w2583
                      frame 1, Default {
                        n3215 = local read "玩家一財產"() -> (w2612:dbl)
                      }
                      frame 2 {
                        n3216 = local read "玩家二財產"() -> (w2613:dbl)
                      }
                      frame 3 {
                        n3217 = local read "玩家三財產"() -> (w2614:dbl)
                      }
                      frame 4 {
                        n3218 = local read "玩家四財產"() -> (w2615:dbl)
                      }
                    }
                    n3219 = call "各種價格.vi"("Numeric"=w2584) -> ("買空地"=w2582:dbl)  [unwired: 4 in, 5 out]
                    n3220 = Greater Or Equal?(x=w2583, y=w2582) -> (x >= y?=w2581:bool)
                    n3221 = case shown="True" w2581 {
                      tunnel: w2584 -> [_ w2586]
                      frame False {
                        # "錢不夠"
                        n3222 = call "錢不夠.vi"() -> ()  [unwired: 4 in]
                      }
                      frame True {
                        # "錢夠"
                        n3223 = local read "換誰?"() -> (w2587:dbl)
                        n3224 = case shown="1, Default" w2587 {
                          selector: w2587 -> [w2591 w2597 w2603 w2609]
                          tunnel: w2586 -> [w2590 w2596 w2602 w2608]
                          frame 1, Default {
                            # "誰買了地"
                            n3225 = call "各種價格.vi"("Numeric"=w2590) -> ("買空地"=w2589:dbl)  [unwired: 4 in, 5 out]
                            n3226 = local read "玩家一財產"() -> (w2593:dbl)
                            n3227 = Subtract(x=w2593, y=w2589) -> (x-y=w2592:dbl)
                            n3228 = local write "玩家一財產"(w2592) -> ()
                            n3229 = call "數字轉顏色.vi"("數字"=w2591) -> ("顏色數字"=w2588:dbl)  [unwired: 2 in]
                            n3230 = local write "22阿里山"(w2588) -> ()
                            n3231 = local write "阿里山所有"(w2588) -> ()
                          }
                          frame 2 {
                            # "誰買了地"
                            n3232 = call "各種價格.vi"("Numeric"=w2596) -> ("買空地"=w2595:dbl)  [unwired: 4 in, 5 out]
                            n3233 = local read "玩家二財產"() -> (w2599:dbl)
                            n3234 = Subtract(x=w2599, y=w2595) -> (x-y=w2598:dbl)
                            n3235 = local write "玩家二財產"(w2598) -> ()
                            n3236 = call "數字轉顏色.vi"("數字"=w2597) -> ("顏色數字"=w2594:dbl)  [unwired: 2 in]
                            n3237 = local write "22阿里山"(w2594) -> ()
                            n3238 = local write "阿里山所有"(w2594) -> ()
                          }
                          frame 3 {
                            # "誰買了地"
                            n3239 = local read "玩家三財產"() -> (w2604:dbl)
                            n3240 = call "各種價格.vi"("Numeric"=w2602) -> ("買空地"=w2601:dbl)  [unwired: 4 in, 5 out]
                            n3241 = Subtract(x=w2604, y=w2601) -> (x-y=w2605:dbl)
                            n3242 = call "數字轉顏色.vi"("數字"=w2603) -> ("顏色數字"=w2600:dbl)  [unwired: 2 in]
                            n3243 = local write "玩家三財產"(w2605) -> ()
                            n3244 = local write "22阿里山"(w2600) -> ()
                            n3245 = local write "阿里山所有"(w2600) -> ()
                          }
                          frame 4 {
                            # "誰買了地"
                            n3246 = call "各種價格.vi"("Numeric"=w2608) -> ("買空地"=w2607:dbl)  [unwired: 4 in, 5 out]
                            n3247 = local read "玩家四財產"() -> (w2611:dbl)
                            n3248 = Subtract(x=w2611, y=w2607) -> (x-y=w2610:dbl)
                            n3249 = local write "玩家四財產"(w2610) -> ()
                            n3250 = call "數字轉顏色.vi"("數字"=w2609) -> ("顏色數字"=w2606:dbl)  [unwired: 2 in]
                            n3251 = local write "22阿里山"(w2606) -> ()
                            n3252 = local write "阿里山所有"(w2606) -> ()
                          }
                        }
                      }
                    }
                  }
                }
              }
            }
          }
          frame 23 {
            n3253 = local read "嘉義縣所有"() -> (w2616:u32)
            n3254 = Equal?(x=w2616, y=u32 16777215) -> (x = y?=w2619:bool)
            n3255 = case shown="True" w2619 {
              tunnel: w2618 -> [w2642 w2680]
              tunnel: [w2632 FALSE] -> w2617
              frame False {
                # "有主地"
                n3256 = local read "換誰?"() -> (w2635:dbl)
                n3257 = local read "嘉義縣所有"() -> (w2622:u32)
                n3258 = call "數字轉顏色.vi"("數字"=w2635) -> ("顏色數字"=w2646:dbl)  [unwired: 2 in]
                n3259 = case shown="4" w2635 {
                  tunnel: [w2675 w2676 w2677 w2678] -> w2641
                  frame 1, Default {
                    n3260 = local read "玩家一財產"() -> (w2675:dbl)
